vi "RT Microprocessor.vi"() -> ()   [LabVIEW 2014]
doc: "This is the primary Real-Time VI."
panel:
  in  "Max Temp":fxp<+/-,32,13>=33.0
  out "RPM":fxp<+,32,16>
  out "Temp":fxp<+/-,32,13>
  out "Voltage":fxp<+/-,24,5>
  out "Battery State":enum16{"Charged", "Running", "Low Batt"}(ring)
  out "Temp Warning":bool
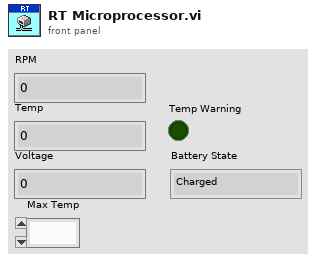
[diagram p1: front panel]
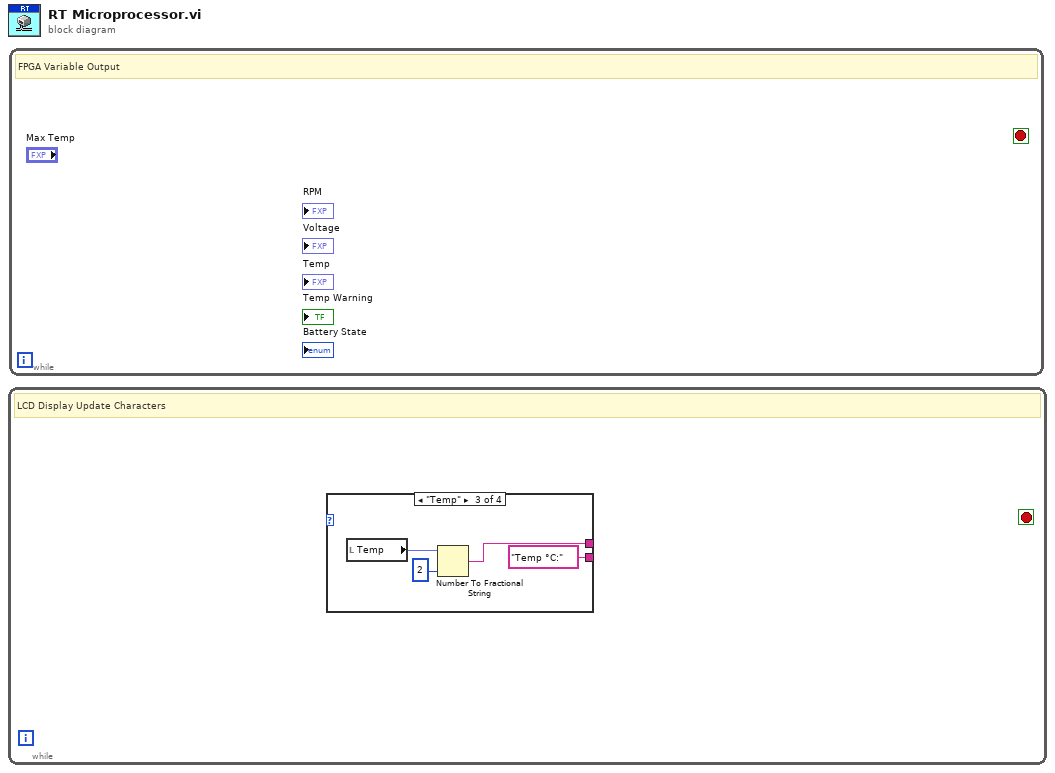
[diagram p0: block diagram]
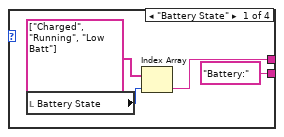
[diagram p2: hidden frame]
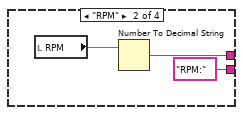
[diagram p3: hidden frame]
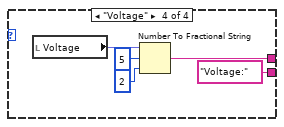
[diagram p4: hidden frame]
diagram:
  n1 = while {
    stop <- _ stop-if-true
    # "LCD Display Update Characters"
    n2 = case shown="\"Temp\"" {
      selector: _ -> [_ _ _ _]
      tunnel: ["Battery:" "RPM:" "Temp °C:" "Voltage:"] -> _
      tunnel: [w3 w6 w9 w14] -> _
      frame "Battery State" {
        n3 = local read "Battery State"() -> (w2:enum16{"Charged", "Running", "Low Batt"})
        n4 = Index Array(array=string[] ["Charged", "Running", "Low Batt"], index=w2) -> (element=w3:string)
      }
      frame "RPM" {
        n5 = local read "RPM"() -> (w5:fxp<+,32,16>)
        n6 = Number To Decimal String(number=w5) -> (decimal integer string=w6:string)  [unwired: 1 in]
      }
      frame "Temp" {
        n7 = local read "Temp"() -> (w8:fxp<+/-,32,13>)
        n8 = Number To Fractional String(number=w8, precision (6)=i16 2) -> (F-format string=w9:string)  [unwired: 2 in]
      }
      frame "Voltage" {
        n9 = local read "Voltage"() -> (w12:fxp<+/-,24,5>)
        n10 = Number To Fractional String(number=w12, width (-)=i16 5, precision (6)=i16 2) -> (F-format string=w14:string)  [unwired: 1 in]
      }
    }
  }
  n11 = while {
    stop <- _ stop-if-true
    # "FPGA Variable Output"
  }
